vi "DAC upload.vi"(7 "dt":dbl=2e-06, 8 "error in":errorcluster, 9 "voltage":dbl[][](array[numeric]), 10 "time":dbl[](array[numeric]), 11 "device":tag) -> (0 "error out":errorcluster, 2 "clock":refnum<k21>, 3 "output":refnum<k21>)   [LabVIEW 2012]
uses:
  <vilib>/DAQmx/write.llb/DAQmx Write (Analog 1D Wfm NChan NSamp).vi
  <vilib>/DAQmx/create/channels.llb/DAQmx Create Channel (AO-Voltage-Basic).vi
  <vilib>/DAQmx/configure/timing.llb/DAQmx Timing (Sample Clock).vi
  <vilib>/DAQmx/create/channels.llb/DAQmx Create Channel (CO-Pulse Generation-Frequency).vi
  <vilib>/DAQmx/configure/timing.llb/DAQmx Timing (Implicit).vi
  <vilib>/DAQmx/configure/trigger.llb/DAQmx Start Trigger (Digital Edge).vi
  <vilib>/DAQmx/miscellaneous.llb/DAQmx Fill In Error Info.vi
  <vilib>/regexp/Match Regular Expression.xnode
  <resource>/objmgr/daqmx.rc
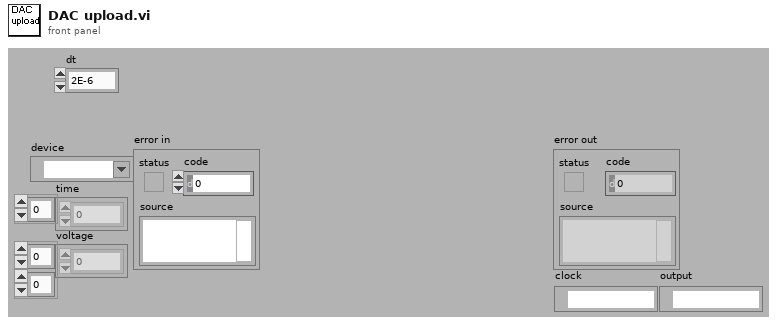
[diagram p1: front panel]
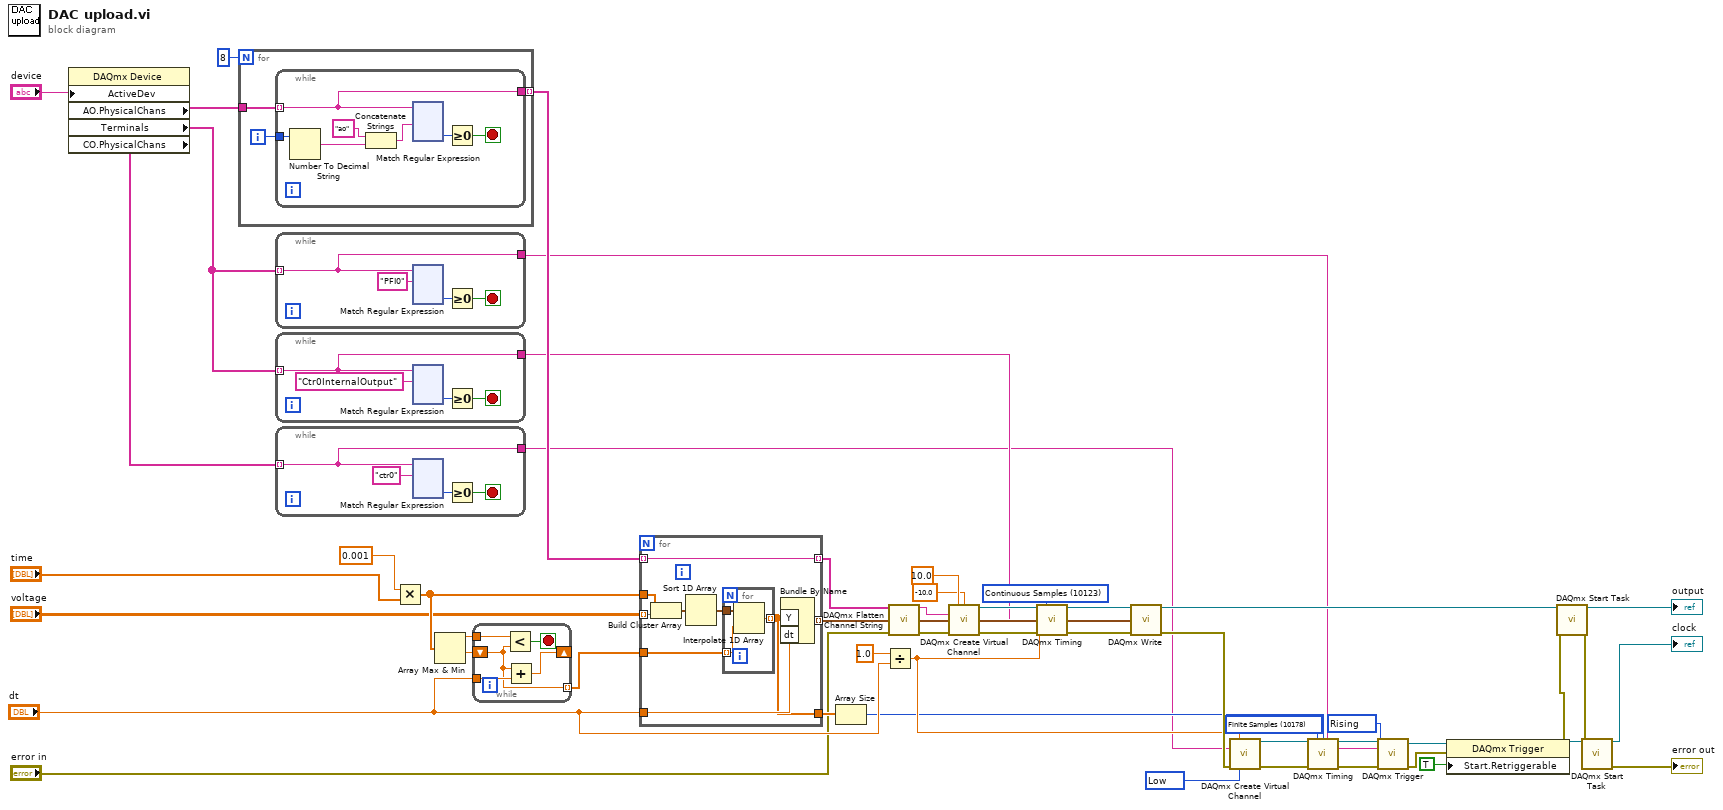
[diagram p0: block diagram]
diagram:
  w31 = 10214 items=["High"=10192, "Low"=10214] ("idle state")
  w32 = 10280 items=["Rising"=10280, "Falling"=10171] ("edge")
  w38 = 10178 items=["Finite Samples"=10178, "Continuous Samples"=10123, "Hardware Timed Single Point"=12522] ("sample mode")
  w44 = 10123 items=["Finite Samples"=10178, "Continuous Samples"=10123, "Hardware Timed Single Point"=12522] ("sample mode")
  n1 = property class="DAQmx Device"("ActiveDev"="device") -> ("AO.PhysicalChans"=w9:tag[], "Terminals"=w7:tag[], "CO.PhysicalChans"=w6:tag[])  [unwired: 2 in, 2 out]
  n2 = for {
    N: 8 -> [_]
    tunnel: w9 -> [w54]
    tunnel: [w52] -> w5 mode=indexing
    i -> [w53]
    n3 = while {
      tunnel: w54 -> [w58] mode=indexing
      tunnel: w53 -> [w61]
      tunnel: [w58] -> w52
      stop <- w59 stop-if-true
      n4 = Number To Decimal String(number=w61) -> (decimal integer string=w57:string)  [unwired: 1 in]
      n5 = Concatenate Strings("ao" ("string"), w57) -> (w55:string)
      n6 = xnode "Match Regular Expression"("input string"=w58, "regular expression"=w55) -> ("offset past match"=w60:i32)  [unwired: 4 in, 4 out]
      n7 = Greater Or Equal To 0?(x=w60) -> (x >= 0?=w59:bool)
    }
  }
  n8 = while {
    tunnel: w7 -> [w174] mode=indexing
    tunnel: [w174] -> w2
    stop <- w175 stop-if-true
    n9 = xnode "Match Regular Expression"("input string"=w174, "regular expression"="PFI0" ("string")) -> ("offset past match"=w176:i32)  [unwired: 4 in, 4 out]
    n10 = Greater Or Equal To 0?(x=w176) -> (x >= 0?=w175:bool)
  }
  n11 = while {
    tunnel: w7 -> [w289] mode=indexing
    tunnel: [w289] -> w4
    stop <- w290 stop-if-true
    n12 = xnode "Match Regular Expression"("input string"=w289, "regular expression"="Ctr0InternalOutput" ("string")) -> ("offset past match"=w291:i32)  [unwired: 4 in, 4 out]
    n13 = Greater Or Equal To 0?(x=w291) -> (x >= 0?=w290:bool)
  }
  n14 = while {
    tunnel: w6 -> [w404] mode=indexing
    tunnel: [w404] -> w3
    stop <- w405 stop-if-true
    n15 = xnode "Match Regular Expression"("input string"=w404, "regular expression"="ctr0" ("string")) -> ("offset past match"=w406:i32)  [unwired: 4 in, 4 out]
    n16 = Greater Or Equal To 0?(x=w406) -> (x >= 0?=w405:bool)
  }
  n17 = Multiply(x=0.001, y="time") -> (x*y=w21:dbl[])
  n18 = Array Max & Min(array=w21) -> (max value=w19:dbl, min value=w17:dbl)  [unwired: 2 out]
  n19 = while {
    tunnel: [w518] -> w20 mode=indexing
    shift-right: [w520] -> _
    shift-left: w17 -> [w518]
    tunnel: w19 -> [w522]
    tunnel: "dt" -> [w519]
    stop <- w521 stop-if-true
    n20 = Less?(x=w522, y=w518) -> (x < y?=w521:bool)
    n21 = Add(x=w518, y=w519) -> (x+y=w520:dbl)
  }
  n22 = for {
    tunnel: "voltage" -> [w531] mode=indexing
    tunnel: w21 -> [w530]
    tunnel: w20 -> [w529]
    tunnel: [w528] -> w49 mode=indexing
    tunnel: "dt" -> [w525]
    tunnel: [w524] -> w50
    tunnel: w5 -> [w523] mode=indexing
    tunnel: [w523] -> w16 mode=indexing
    n23 = Build Cluster Array(w530, w531) -> (w526:cluster{dbl, "Voltage":dbl}[])
    n24 = Sort 1D Array(array=w526) -> (sorted array=w527:cluster{dbl, "Voltage":dbl}[])
    n25 = for {
      tunnel: w527 -> [w534]
      tunnel: w529 -> [w533] mode=indexing
      tunnel: [w532] -> w524 mode=indexing
      n26 = Interpolate 1D Array(1:w533, 2:w534) -> (0:w532:dbl)
    }
    n27 = Bundle By Name("Y"=w524, "dt"=w525) -> (w528:waveform(dbl))  [unwired: 1 in]
  }
  n28 = Array Size(array=w50) -> (size(s)=w25:i32)
  n29 = Divide(x=1.0, y="dt") -> (x/y=w26:dbl)
  n30 = call <vilib>:"DAQmx Flatten Channel String.vi"("names in"=w16, "error in"="error in") -> ("names out"=w47:string, "error out"=w48:errorcluster)  [unwired: 12 in]
  n31 = call-poly <vilib>:"DAQmx Create Virtual Channel.vi"("maximum value"=10.0, "minimum value"=-10.0, "physical channels"=w47, "error in"=w48) -> ("task out"=w46:refnum<k21>, "error out"=w45:errorcluster)  [unwired: 10 in]
  n32 = call-poly <vilib>:"DAQmx Timing.vi"("task/channels in"=w46, "sample mode"=w44, "rate"=w26, "source"=w4, "error in"=w45) -> ("task out"=w36:refnum<k21>, "error out"=w37:errorcluster)  [unwired: 9 in]
  n33 = call-poly <vilib>:"DAQmx Write.vi"("task/channels in"=w36, "data"=w49, "error in"=w37) -> ("task out"=w29:refnum<k21>, "error out"=w35:errorcluster)  [unwired: 10 in, 1 out]
  n34 = call-poly <vilib>:"DAQmx Create Virtual Channel.vi"("frequency"=w26, "counter"=w3, "error in"=w35, "idle state"=w31) -> ("task out"=w42:refnum<k21>, "error out"=w41:errorcluster)  [unwired: 10 in]
  n35 = call-poly <vilib>:"DAQmx Timing.vi"("task/channels in"=w42, "sample mode"=w38, "samples per channel"=w25, "error in"=w41) -> ("task out"=w40:refnum<k21>, "error out"=w39:errorcluster)  [unwired: 10 in]
  n36 = call-poly <vilib>:"DAQmx Trigger.vi"("task/channels in"=w40, "source"=w2, "edge"=w32, "error in"=w39) -> ("task out"=w34:refnum<k21>, "error out"=w33:errorcluster)  [unwired: 10 in]
  n37 = property class="DAQmx Trigger"(reference=w34, error in=w33, "Start.Retriggerable"=TRUE) -> (reference out=w30:refnum<k21>, error out=w28:errorcluster)
  n38 = call <vilib>:"DAQmx Start Task.vi"("task/channels in"=w29, "error in"=w28) -> ("task out"=→"output":refnum<k21>, "error out"=w27:errorcluster)  [unwired: 12 in]
  n39 = call <vilib>:"DAQmx Start Task.vi"("task/channels in"=w30, "error in"=w27) -> ("task out"=→"clock":refnum<k21>, "error out"=→"error out":errorcluster)  [unwired: 12 in]
